vi "Acquisition Message Loop.vi"(8 "error in (no error)":errorcluster caption="错误输入（无错误）", 9 "Angle Data Queue":refnum<queue> caption="角度数据队列", 10 "Analog Data Queue":refnum<queue> caption="模拟数据队列", 11 "Message Queues":T1 caption="消息队列") -> (0 "error out":errorcluster caption="错误输出")   [LabVIEW 2015, in "Acquisition.lvlib"]
doc: "该消息循环负责处理硬件数据采集的相关消息。"
uses:
  Acquisition.lvlib
  support/Message Queue/All Message Queues.ctl
  support/Message Queue/Message Cluster.ctl
  Hardware Configuration.ctl
  Acquisition State.ctl
  support/Message Queue/Enqueue Message (Single).vi
  <vilib>/Utility/error.llb/Error Cluster From Error Code.vi
  <vilib>/ErrorRing/Error Ring.xnode
  support/Message Queue/Message Queue.lvlib
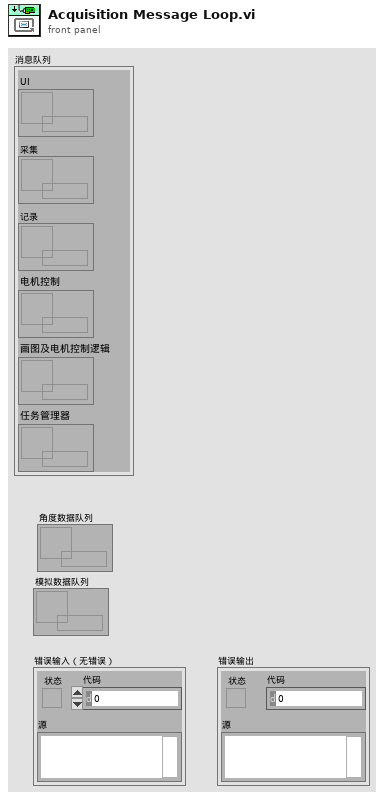
[diagram p1: front panel]
types:
  T1 = typedef "Message Queue.lvlib/All Message Queues.ctl" = cluster{"UI":refnum<queue>, "Acquisition":refnum<queue>, "Logging":refnum<queue>, "plot logic":refnum<queue>, "Action Control":refnum<queue>, "TaskMan":refnum<queue>}
  T2 = typedef "Acquisition.lvlib/Hardware Configuration.ctl" = cluster{"电压读取设置":cluster{"DAQmx Channel":tag, "Max Input":dbl, "Min Input":dbl, "Sample Rate":dbl, "Sample Number":i32, "DAQmx Task":refnum<k21>, "device in":tag}, "角度传感器设置":cluster{"counter":tag, "units":i32, "分辨率":i32, "初始角度":dbl, "DecodingType":i32, "A相端口":tag, "B相端口":tag, "task in":refnum<k21>}}
  T3 = typedef "Acquisition.lvlib/Acquisition State.ctl" = enum16{"Idle", "Acquiring"}
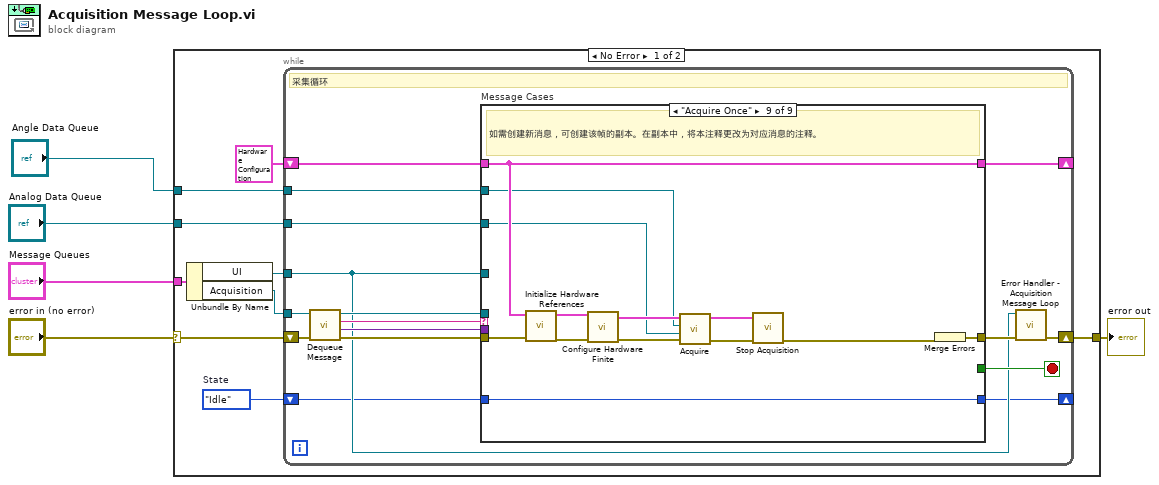
[diagram p0: block diagram]
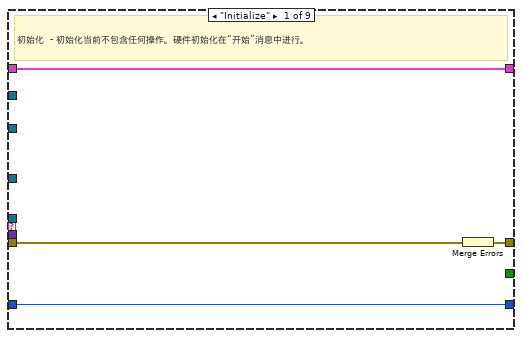
[diagram p2: hidden frame]
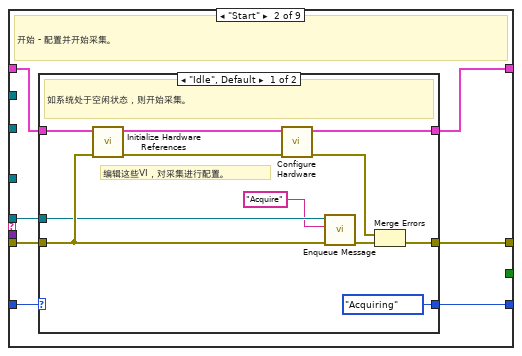
[diagram p3: hidden frame]
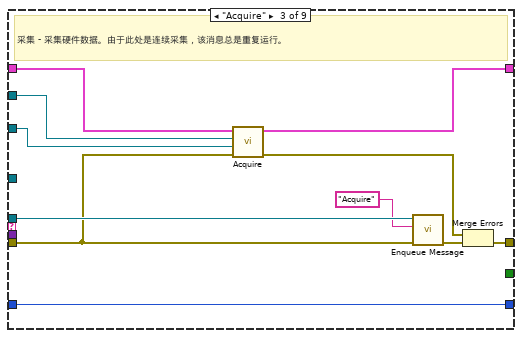
[diagram p5: hidden frame]
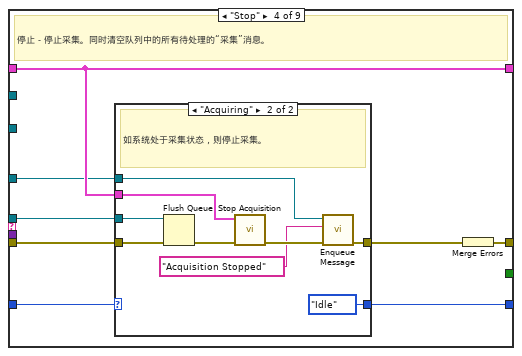
[diagram p6: hidden frame]
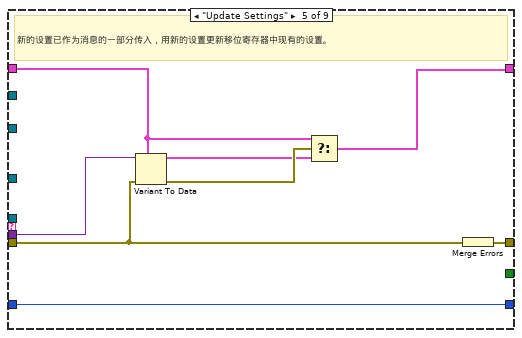
[diagram p8: hidden frame]
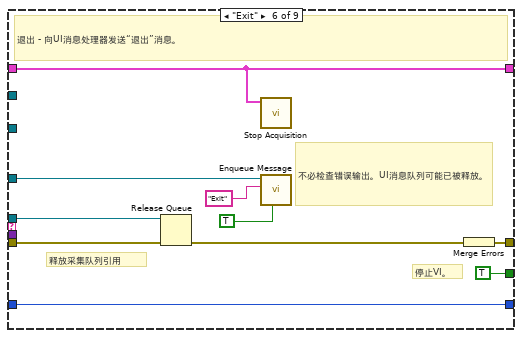
[diagram p9: hidden frame]
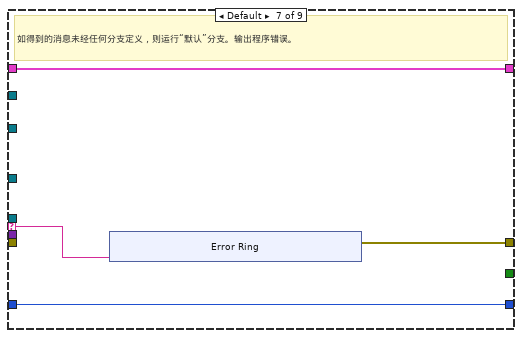
[diagram p10: hidden frame]
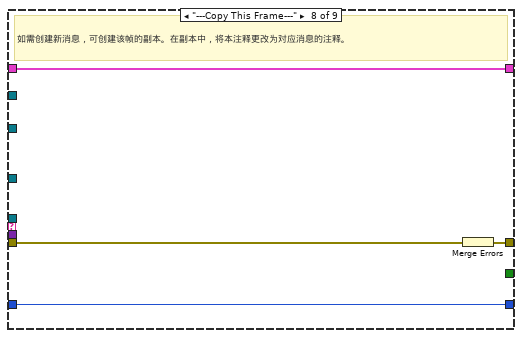
[diagram p11: hidden frame]
diagram:
  n1 = case shown="No Error" "error in (no error)" {
    selector: "error in (no error)" -> [w10 w132]
    tunnel: "Message Queues" -> [w14 _]
    tunnel: [w12 w132] -> w4
    tunnel: "Angle Data Queue" -> [w8 _]
    tunnel: "Analog Data Queue" -> [w7 _]
    frame No Error {
      w6 = Acquisition_State."Idle"  # State
      n2 = Unbundle By Name(w14) -> ("UI"=w9:refnum<queue>, "Acquisition"=w13:refnum<queue>)
      n3 = while {
        tunnel: w13 -> [w22]
        shift-right: [w29] -> _
        shift-left: T2 {"电压读取设置"={"DAQmx Channel"="", "Max Input"=0.0, "Min Input"=0.0, "Sample Rate"=0.0, "Sample Number"=0, "DAQmx Task"="", "device in"=""}, "角度传感器设置"={"counter"="Dev1/ctr0", "units"=10146, "分辨率"=0, "初始角度"=0.0, "DecodingType"=10092, "A相端口"="/Dev1/PFI8", "B相端口"="/Dev1/PFI8", "task in"=""}} ("Data Cluster") -> [w30]
        shift-right: [w18] -> w12
        shift-left: w10 -> [w27]
        tunnel: w9 -> [w17]
        tunnel: w8 -> [w21]
        tunnel: w7 -> [w20]
        shift-right: [w15] -> _
        shift-left: w6 -> [w16]
        stop <- w28 stop-if-true
        # "采集循环"
        n4 = call "Dequeue Message.vi"("error in (no error)"=w27, "Message Queue"=w22) -> ("error out"=w26:errorcluster, "Message Data"=w24:variant, "Message"=w25:string, "dup Message Queue"=w23:refnum<queue>)  [unwired: 6 in]
        n5 = case "Message Cases" shown="\"Acquire Once\"" w25 {
          selector: w25 -> [_ _ _ _ _ _ w106 _ _]
          tunnel: w23 -> [_ w38 w64 w71 _ w96 _ _ _]
          tunnel: w26 -> [w33 w39 w63 w73 w87 w100 _ w118 w127]
          tunnel: [w34 w41 w66 w74 w93 w102 w105 w116 w131] -> w19
          tunnel: w30 -> [w32 w40 w60 w72 w89 w95 w107 w117 w126]
          tunnel: [w32 w37 w61 w72 w88 w95 w107 w117 w126] -> w29
          tunnel: [_ _ _ _ _ TRUE _ _ _] -> w28
          tunnel: w24 -> [_ _ _ _ w92 _ _ _ _]
          tunnel: w17 -> [_ _ _ w70 _ w101 _ _ _]
          tunnel: w21 -> [_ _ w58 _ _ _ _ _ w123]
          tunnel: w20 -> [_ _ w57 _ _ _ _ _ w122]
          tunnel: w16 -> [w31 w36 w56 w69 w86 w94 w104 w115 w130]
          tunnel: [w31 w35 w56 w68 w86 w94 w104 w115 w130] -> w15
          frame "Initialize" {
            # "初始化  - 初始化当前不包含任何操作。硬件初始化在“开始”消息中进行。"
            n6 = Merge Errors(w33) -> (w34:errorcluster)
          }
          frame "Start" {
            # "开始 - 配置并开始采集。"
            n7 = case shown="\"Idle\", Default" w36 {
              selector: w36 -> [_ w53]
              tunnel: [w52 w55] -> w41
              tunnel: w40 -> [w51 w54]
              tunnel: w39 -> [w50 w55]
              tunnel: w38 -> [w48 _]
              tunnel: [w44 w54] -> w37
              tunnel: [Acquisition_State."Acquiring" ("State") w53] -> w35
              frame "Idle", Default {
                # "编辑这些VI，对采集进行配置。"
                # "如系统处于空闲状态，则开始采集。"
                n8 = call "Initialize Hardware References.vi"("error in (no error)"=w50, "Hardware Resources in"=w51) -> ("error out"=w47:errorcluster, "Hardware Resources out"=w45:T2)  [unwired: 8 in]
                n9 = call "Configure Hardware.vi"("error in (no error)"=w47, "Hardware Resources in"=w45) -> ("error out"=w46:errorcluster, "Hardware Resources out"=w44:T2)  [unwired: 8 in]
                n10 = call-poly "Enqueue Message.vi"("error in (no error)"=w50, "Message"="Acquire", "Message Queue"=w48) -> ("error out"=w49:errorcluster)  [unwired: 7 in, 1 out]
                n11 = Merge Errors(w46, w49) -> (w52:errorcluster)
              }
              frame "Acquiring" {
                # "系统已开始采集。忽略“开始”消息。"
              }
            }
          }
          frame "Acquire" {
            # "采集 - 采集硬件数据。由于此处是连续采集，该消息总是重复运行。"
            n12 = call "Acquire.vi"("error in (no error)"=w63, "Analog Data Queue"=w57, "Angle Data Queue"=w58, "Hardware Resources in"=w60) -> ("error out"=w62:errorcluster, "Hardware Resources out"=w61:T2)  [unwired: 6 in]
            n13 = call-poly "Enqueue Message.vi"("error in (no error)"=w63, "Message"="Acquire", "Message Queue"=w64) -> ("error out"=w65:errorcluster)  [unwired: 7 in, 1 out]
            n14 = Merge Errors(w62, w65) -> (w66:errorcluster)
          }
          frame "Stop" {
            # "停止－停止采集。同时清空队列中的所有待处理的“采集”消息。"
            n15 = case shown="\"Acquiring\"" w69 {
              selector: w69 -> [w76 _]
              tunnel: w73 -> [w75 w85]
              tunnel: w72 -> [_ w84]
              tunnel: w71 -> [_ w82]
              tunnel: w70 -> [_ w81]
              tunnel: [w76 Acquisition_State."Idle" ("State")] -> w68
              tunnel: [w75 w79] -> w67
              frame "Idle", Default {
                # "系统已处于空闲状态。忽略“停止”消息。"
              }
              frame "Acquiring" {
                # "如系统处于采集状态，则停止采集。"
                n16 = Flush Queue(queue=w82, error in (no error)=w85) -> (error out=w83:errorcluster)  [unwired: 2 out]
                n17 = call "Stop Acquisition.vi"("error in (no error)"=w83, "Hardware Resources in"=w84) -> ("error out"=w80:errorcluster)  [unwired: 9 in]
                n18 = call-poly "Enqueue Message.vi"("error in (no error)"=w80, "Message"="Acquisition Stopped", "Message Queue"=w81) -> ("error out"=w79:errorcluster)  [unwired: 7 in, 1 out]
              }
            }
            n19 = Merge Errors(w67) -> (w74:errorcluster)
          }
          frame "Update Settings" {
            # "新的设置已作为消息的一部分传入，用新的设置更新移位寄存器中现有的设置。"
            n20 = Variant To Data(error in=w87, type=w89, Variant=w92) -> (data=w90:T2, error out=w91:errorcluster)
            n21 = Select(t=w89, s=w91, f=w90) -> (s? t:f=w88:T2)
            n22 = Merge Errors(w87) -> (w93:errorcluster)
          }
          frame "Exit" {
            # "不必检查错误输出。UI消息队列可能已被释放。"
            # "释放采集队列引用"
            # "停止VI。"
            # "退出 - 向UI消息处理器发送“退出”消息。"
            n23 = Release Queue(queue=w96, error in (no error)=w100) -> (error out=w97:errorcluster)  [unwired: 1 in, 2 out]
            n24 = call "Stop Acquisition.vi"("Hardware Resources in"=w95) -> ()  [unwired: 10 in, 1 out]
            n25 = call-poly "Enqueue Message.vi"("Priority Message? (F)"=TRUE, "Message"="Exit", "Message Queue"=w101) -> ()  [unwired: 7 in, 2 out]
            n26 = Merge Errors(w97) -> (w102:errorcluster)
          }
          frame Default {
            # "如得到的消息未经任何分支定义，则运行“默认”分支。输出程序错误。"
            n27 = xnode "Error Ring"("parameter 0"=w106) -> ("error out"=w105:errorcluster)
          }
          frame "---Copy This Frame---" {
            # "如需创建新消息，可创建该帧的副本。在副本中，将本注释更改为对应消息的注释。"
            n28 = Merge Errors(w118) -> (w116:errorcluster)
          }
          frame "Acquire Once" {
            # "如需创建新消息，可创建该帧的副本。在副本中，将本注释更改为对应消息的注释。"
            n29 = call "Initialize Hardware References.vi"("error in (no error)"=w127, "Hardware Resources in"=w126) -> ("error out"=w128:errorcluster, "Hardware Resources out"=w129:T2)  [unwired: 8 in]
            n30 = call "Configure Hardware Finite.vi"("error in (no error)"=w128, "Hardware Resources in"=w129) -> ("error out"=w125:errorcluster, "Hardware Resources out"=w124:T2)  [unwired: 8 in]
            n31 = call "Acquire.vi"("error in (no error)"=w125, "Analog Data Queue"=w122, "Angle Data Queue"=w123, "Hardware Resources in"=w124) -> ("error out"=w121:errorcluster, "Hardware Resources out"=w120:T2)  [unwired: 6 in]
            n32 = call "Stop Acquisition.vi"("error in (no error)"=w121, "Hardware Resources in"=w120) -> ("error out"=w119:errorcluster)  [unwired: 9 in]
            n33 = Merge Errors(w119) -> (w131:errorcluster)
          }
        }
        n34 = call "Error Handler - Acquisition Message Loop.vi"("error in (no error)"=w19, "Message Queue"=w17) -> ("dup error in"=w18:errorcluster)  [unwired: 8 in, 1 out]
      }
    }
    frame Error {
    }
  }
  "error out" <- w4
